vi "Spark MAX Get Cached Parameter.vi"(8 "error in (no error)":errorcluster, 10 "Parameter ID":T3, 11 "SPARK MAX Device Ref in":T1={"Ext ID"=0, "Status 0 Session Handle"=0, "Status 1 Session Handle"=0, "Param Session Handle"=0, "Param Cache ref"=refnum, "CAN Timeout"=0, "Status 2 Session Handle"=0, "Status 3 Session Handle"=0, "Inverted No WPILib"=FALSE, "Has Configured Limit Sw"=FALSE, "Has Configured Alt Encoder"=FALSE, "Status 4 Session Handle"=0, "SPARK Model"=enum."Unknown", "Max CAN Retries"=5, "CAN Timeout (ms)"=20}) -> (0 "error out":errorcluster, 1 "Parameter Type":T4=enum."Signed Int", 2 "Parameter Raw":u32, 3 "found":bool, 5 "Timestamp":u32)   [LabVIEW 2023]
uses:
  Typedef/Spark MAX Parameter Type.ctl
  Typedef/Spark MAX Parameter Cache Element.ctl
  Typedef/Spark MAX Parameter Status.ctl
  Typedef/SPARK Parameter ID.ctl
  Typedef/Spark MAX Variant Data.ctl
  Typedef/SPARK Model.ctl
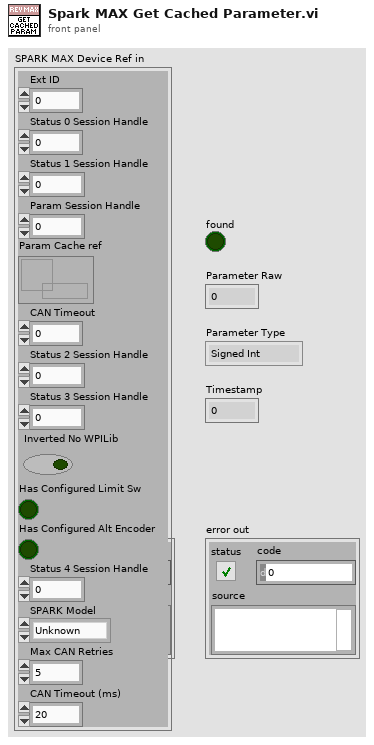
[diagram p1: front panel]
types:
  T1 = typedef "Spark MAX Variant Data.ctl" = cluster{"Ext ID":u32, "Status 0 Session Handle":u32, "Status 1 Session Handle":u32, "Param Session Handle":u32, "Param Cache ref":refnum<data-value>, "CAN Timeout":u32, "Status 2 Session Handle":u32, "Status 3 Session Handle":u32, "Inverted No WPILib":bool, "Has Configured Limit Sw":bool, "Has Configured Alt Encoder":bool, "Status 4 Session Handle":u32, "SPARK Model":T2, "Max CAN Retries":i32, "CAN Timeout (ms)":i32}
  T2 = typedef "SPARK Model.ctl" = enum16{"SPARK MAX", "SPARK Flex", "Unknown"}
  T3 = typedef "SPARK Parameter ID.ctl" = enum16{"kCanID", "kInputMode", "kMotorType", "kCommAdvance", "kSensorType", "kCtrlType", "kIdleMode", "kInputDeadband", "kLegacyFeedbackSensorPID0", "kClosedLoopControlSensor", "kPolePairs", "kCurrentChop", "kCurrentChopCycles", "kP_0", "kI_0", "kD_0", "kF_0", "kIZone_0", "kDFilter_0", "kOutputMin_0", "kOutputMax_0", "kP_1", "kI_1", "kD_1", "kF_1", "kIZone_1", "kDFilter_1", "kOutputMin_1", "kOutputMax_1", "kP_2", "kI_2", "kD_2", "kF_2", "kIZone_2", "kDFilter_2", "kOutputMin_2", "kOutputMax_2", "kP_3", "kI_3", "kD_3", "kF_3", "kIZone_3", "kDFilter_3", "kOutputMin_3", "kOutputMax_3", "kInverted", "kOutputRatio", "kSerialNumberLow", "kSerialNumberMid", "kSerialNumberHigh", "kLimitSwitchFwdPolarity", "kLimitSwitchRevPolarity", "kHardLimitFwdEn", "kHardLimitRevEn", "kSoftLimitFwdEn", "kSoftLimitRevEn", "kRampRate", "kFollowerID", "kFollowerConfig", "kSmartCurrentStallLimit", "kSmartCurrentFreeLimit", "kSmartCurrentConfig", "kSmartCurrentReserved", "kMotorKv", "kMotorR", "kMotorL", "kMotorRsvd1", "kMotorRsvd2", "kMotorRsvd3", "kEncoderCountsPerRev", "kEncoderAverageDepth", "kEncoderSampleDelta", "kEncoderInverted", "kEncoderRsvd1", "kClosedLoopVoltageMode", "kCompensatedNominalVoltage", "kSmartMotionMaxVelocity_0", "kSmartMotionMaxAccel_0", "kSmartMotionMinVelOutput_0", "kSmartMotionAllowedClosedLoopError_0", "kSmartMotionAccelStrategy_0", "kSmartMotionMaxVelocity_1", "kSmartMotionMaxAccel_1", "kSmartMotionMinVelOutput_1", "kSmartMotionAllowedClosedLoopError_1", "kSmartMotionAccelStrategy_1", "kSmartMotionMaxVelocity_2", "kSmartMotionMaxAccel_2", "kSmartMotionMinVelOutput_2", "kSmartMotionAllowedClosedLoopError_2", "kSmartMotionAccelStrategy_2", "kSmartMotionMaxVelocity_3", "kSmartMotionMaxAccel_3", "kSmartMotionMinVelOutput_3", "kSmartMotionAllowedClosedLoopError_3", "kSmartMotionAccelStrategy_3", "kIMaxAccum_0", "kSlot3Placeholder1_0", "kSlot3Placeholder2_0", "kSlot3Placeholder3_0", "kIMaxAccum_1", "kSlot3Placeholder1_1", "kSlot3Placeholder2_1", "kSlot3Placeholder3_1", "kIMaxAccum_2", "kSlot3Placeholder1_2", "kSlot3Placeholder2_2", "kSlot3Placeholder3_2", "kIMaxAccum_3", "kSlot3Placeholder1_3", "kSlot3Placeholder2_3", "kSlot3Placeholder3_3", "kPositionConversionFactor", "kVelocityConversionFactor", "kClosedLoopRampRate", "kSoftLimitFwd", "kSoftLimitRev", "kSoftLimitRsvd0", "kSoftLimitRsvd1", "kAnalogPositionConversion", "kAnalogVelocityConversion", "kAnalogAverageDepth", "kAnalogSensorMode", "kAnalogInverted", "kAnalogSampleDelta", "kAnalogRsvd0", "kAnalogRsvd1", "kDataPortConfig", "kAltEncoderCountsPerRev", "kAltEncoderAverageDepth", "kAltEncoderSampleDelta", "kAltEncoderInverted", "kAltEncoderPositionConversion", "kAltEncoderVelocityConversion", "kAltEncoderRsvd0", "kAltEncoderRsvd1", "kHallSensorSampleRate", "kHallSensorAverageDepth", "kNumParameters", "kDutyCyclePositionFactor", "kDutyCycleVelocityFactor", "kDutyCycleInverted", "kDutyCycleSensorMode", "kDutyCycleAverageDepth", "kDutyCycleSampleDelta", "kDutyCycleOffsetv1p6p2", "kDutyCycleRsvd0", "kDutyCycleRsvd1", "kDutyCycleRsvd2", "kPositionPIDWrapEnable", "kPositionPIDMinInput", "kPositionPIDMaxInput", "kDutyCycleZeroCentered", "kDutyCyclePrescalar", "kDutyCycleOffset", "kProductId", "kDeviceMajorVersion", "kDeviceMinorVersion", "kStatus0Period", "kStatus1Period", "kStatus2Period", "kStatus3Period", "kStatus4Period", "kStatus5Period", "kStatus6Period", "kStatus7Period", "kMAXMotionMaxVelocity_0", "kMAXMotionMaxAccel_0", "kMAXMotionMaxJerk_0", "kMAXMotionAllowedClosedLoopError_0", "kMAXMotionPositionMode_0", "kMAXMotionMaxVelocity_1", "kMAXMotionMaxAccel_1", "kMAXMotionMaxJerk_1", "kMAXMotionAllowedClosedLoopError_1", "kMAXMotionPositionMode_1", "kMAXMotionMaxVelocity_2", "kMAXMotionMaxAccel_2", "kMAXMotionMaxJerk_2", "kMAXMotionAllowedClosedLoopError_2", "kMAXMotionPositionMode_2", "kMAXMotionMaxVelocity_3", "kMAXMotionMaxAccel_3", "kMAXMotionMaxJerk_3", "kMAXMotionAllowedClosedLoopError_3", "kMAXMotionPositionMode_3", "kForceEnableStatus0", "kForceEnableStatus1", "kForceEnableStatus2", "kForceEnableStatus3", "kForceEnableStatus4", "kForceEnableStatus5", "kForceEnableStatus6", "kForceEnableStatus7", "kFollowerModeLeaderId", "kFollowerModeIsInverted", "kDutyCycleEncoderStartPulseUs", "kDutyCycleEncoderEndPulseUs"}
  T4 = typedef "Spark MAX Parameter Type.ctl" = enum16{"Unused", "Signed Int", "Unsigned Int", "Float", "Bool"}
  T5 = typedef "Spark MAX Parameter Status.ctl" = enum16{"Ok", "Invalid Parameter ID", "Mismatch Type", "Access Mode", "Invalid Parameter Value", "Not Implemented/Depcrecated"}
  T6 = typedef "Spark MAX Parameter Cache Element.ctl" = cluster{"Timestamp":u32, "Parameter Raw":u32, "Parameter Type":T4, "Last Access Status":T5}
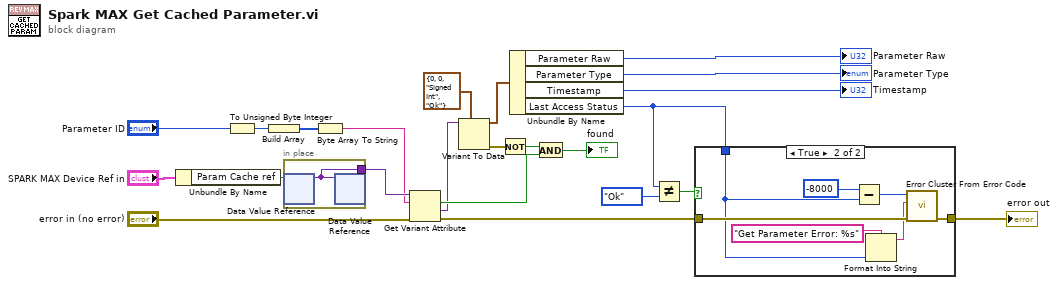
[diagram p0: block diagram]
diagram:
  n1 = Unbundle By Name("SPARK MAX Device Ref in") -> ("Param Cache ref"=w7:refnum<data-value>)
  n2 = To Unsigned Byte Integer(number="Parameter ID") -> (unsigned 8bit integer=w12:u8)
  n3 = Build Array(w12) -> (w10:u8[])
  n4 = in-place {
    in-place-border: [w24] -> w6
    n5 = in-place-dvr #1(w7) -> (w24:variant)  [unwired: 1 out]
    n6 = in-place-dvr #1(w24) -> ()  [unwired: 2 out]
  }
  n7 = Byte Array To String(unsigned byte array=w10) -> (string=w5:string)
  n8 = Get Variant Attribute(Variant=w6, name=w5, error in="error in (no error)") -> (found=w16:bool, value=w14:variant, error out=w19:errorcluster)  [unwired: 1 in, 1 out]
  n9 = Variant To Data(type=T6 {"Timestamp"=0, "Parameter Raw"=0, "Parameter Type"=enum."Signed Int", "Last Access Status"=enum."Ok"} ("Cluster"), Variant=w14) -> (data=w20:T6, error out=w15:errorcluster)  [unwired: 1 in]
  n10 = Not(x=w15) -> (.not. x?=w17:bool)
  n11 = Unbundle By Name(w20) -> ("Parameter Raw"=→"Parameter Raw":u32, "Parameter Type"=→"Parameter Type":T4, "Timestamp"=→"Timestamp":u32, "Last Access Status"=w3:T5)
  n12 = And(x=w17, y=w16) -> (x .and. y?=→"found":bool)
  n13 = Not Equal?(x=w3, y=Spark_MAX_Parameter_Status."Ok") -> (x != y?=w2:bool)
  n14 = case shown="True" w2 {
    tunnel: w19 -> [w25 w32]
    tunnel: [w25 w31] -> w4
    tunnel: w3 -> [_ w28]
    frame False {
    }
    frame True {
      n15 = Subtract(x=-8000 ("error code (0)"), y=w28) -> (x-y=w29:i32)
      n16 = Format Into String(format string="Get Parameter Error: %s", w28) -> (resulting string=w27:string)  [unwired: 2 in, 1 out]
      n17 = call <vilib>:"Error Cluster From Error Code.vi"("error in (no error)"=w32, "error message (\"\")"=w27, "error code (0)"=w29) -> ("error out"=w31:errorcluster)  [unwired: 6 in]
    }
  }
  "error out" <- w4
